vi "Calculate Adjacent Flashes.vi"(9 "Flashes Columns":i32[](array[numeric]), 10 "Flashes Rows":i32[](array[numeric]), 11 "Octopus Energy Matrix In":i32[][](array[numeric])) -> (0 "Flash Count":i32, 3 "Octopus Energy Matrix Out":i32[][](array[numeric]))   [LabVIEW 2019, in "Day 11.lvlib"]
uses:
  Day 11.lvlib
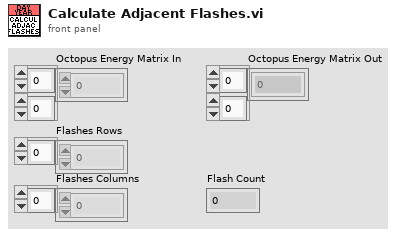
[diagram p1: front panel]
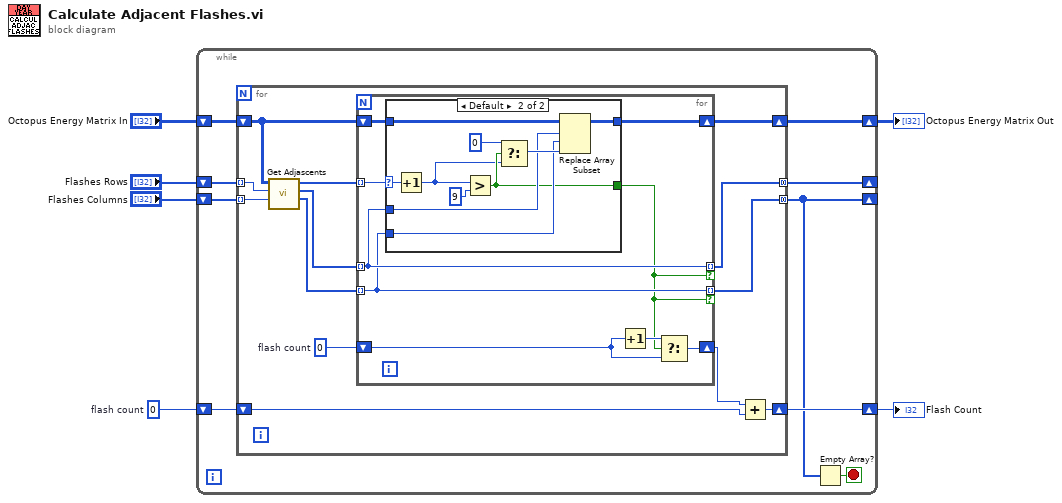
[diagram p0: block diagram]
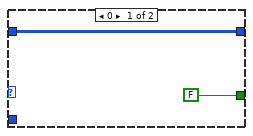
[diagram p2: hidden frame]
diagram:
  w6 = 0  # flash count
  n1 = while {
    shift-right: [w12] -> w3
    shift-left: w6 -> [w15]
    shift-right: [w13] -> w4
    shift-left: "Octopus Energy Matrix In" -> [w14]
    shift-right: [w9] -> _
    shift-left: "Flashes Rows" -> [w11]
    shift-right: [w8] -> _
    shift-left: "Flashes Columns" -> [w10]
    stop <- w7 stop-if-true
    n2 = for {
      shift-right: [w22] -> w13
      shift-left: w14 -> [w24]
      shift-right: [w19] -> w12
      shift-left: w15 -> [w17]
      tunnel: w11 -> [w28] mode=indexing
      tunnel: w10 -> [w27] mode=indexing
      tunnel: [w21] -> w9 mode=concatenating
      tunnel: [w20] -> w8 mode=concatenating
      w23 = 0  # flash count
      n3 = call "Get Adjascents.vi"("Column In"=w27, "Row In"=w28, "Array In"=w24) -> ("Columns Out"=w25:i32[], "Rows Out"=w26:i32[], "Adjacent Elements"=w16:i32[])  [unwired: 6 in]
      n4 = for {
        tunnel: w16 -> [w29] mode=indexing
        tunnel: w26 -> [w32] mode=indexing
        tunnel: w25 -> [w31] mode=indexing
        tunnel: [w32] -> w21 mode=indexing if=w30
        tunnel: [w31] -> w20 mode=indexing if=w30
        shift-right: [w36] -> w22
        shift-left: w24 -> [w37]
        shift-right: [w33] -> w18
        shift-left: w23 -> [w34]
        n5 = case shown="Default" w29 {
          selector: w29 -> [_ w41]
          tunnel: w37 -> [w39 w48]
          tunnel: [w39 w47] -> w36
          tunnel: w32 -> [_ w44]
          tunnel: w31 -> [_ w43]
          tunnel: [FALSE w42] -> w30
          frame 0 {
          }
          frame Default {
            n6 = Increment(x=w41) -> (x+1=w40:i32)
            n7 = Greater?(x=w40, y=9) -> (0:w42:bool)
            n8 = Select(t=0 ("y"), s=w42, f=w40) -> (s? t:f=w45:i32)
            n9 = Replace Array Subset(array=w48, new element=w45, index (row)=w44, index (col)=w43) -> (w47:i32[][])
          }
        }
        n10 = Increment(x=w34) -> (x+1=w35:i32)
        n11 = Select(t=w35, s=w30, f=w34) -> (s? t:f=w33:i32)
      }
      n12 = Add(x=w18, y=w17) -> (x+y=w19:i32)
    }
    n13 = Empty Array?(array=w8) -> (empty?=w7:bool)
  }
  "Octopus Energy Matrix Out" <- w4
  "Flash Count" <- w3
